vi "PathPlanner_Cmd_FollowRamsetePathExecute.vi"(5 "PathPlanner_Cmd_FollowRamConfig":T16={"ControlPastEnd_Sec"=3.0, "ReplanningConfig"={"enableInitialReplanning"=TRUE, "enableDynamicReplanning"=FALSE, "dynamicReplanningTotalErrorThreshold"=1.0, "dynamicReplanningErrorSpikeThreshold"=0.25}, "Trigger Events"=TRUE, "RAMSETE_EXE_TUNING SI"={"B"=2.0, "Zeta"=0.7, "X Tolerance M"=2.0, "Y Tolerance M"=0.7, "Heading Tolerance RAD"=0.7, "Track Width M"=2.0, "Max Speed M/S"=2.0}} {"RAMSETE_EXE_TUNING SI"."Max Speed M/S" format="%13.4f"; "RAMSETE_EXE_TUNING SI"."Track Width M" format="%13.4f"; "RAMSETE_EXE_TUNING SI"."Heading Tolerance RAD" format="%13.4f"; "RAMSETE_EXE_TUNING SI"."Y Tolerance M" format="%13.4f"; "RAMSETE_EXE_TUNING SI"."X Tolerance M" format="%13.4f"; "RAMSETE_EXE_TUNING SI"."Zeta" format="%13.4f"; "RAMSETE_EXE_TUNING SI"."B" format="%13.4f"}, 6 "PassthroughTime_SEC":dbl=-1.0, 7 "PathPlannerPath":T7={"BezierPoints"=[], "PreviewStartingRotation"={"VALUE"=0.0, "COS"=1.0, "SIN"=0.0}, "Reversed"=FALSE, "RotationTargets"=[], "ConstraintZones"=[], "EventMarkers"=[], "GlobalConstraints"={"MaxVelocityMps;"=0.0, "MaxAccelerationMpsSq;"=0.0, "MaxAngularVelRadPsEc;"=0.0, "MaxAngularAccRadPSecSq"=0.0, "Exists"=FALSE}, "GoalEndState"={"Velocity"=0.0, "Rotation"={"VALUE"=0.0, "COS"=1.0, "SIN"=0.0}}, "AllPoints"=[]} {"AllPoints"."HolonomicRotation"."SIN" format="%13.4f"; "AllPoints"."HolonomicRotation"."COS" format="%13.4f"; "AllPoints"."HolonomicRotation"."VALUE" format="%13.4f"; "AllPoints"."Position"."Y" format="%14.3f"; "AllPoints"."Position"."X" format="%14.3f"; "GoalEndState"."Rotation"."SIN" format="%13.4f"; "GoalEndState"."Rotation"."COS" format="%13.4f"; "GoalEndState"."Rotation"."VALUE" format="%13.4f"; "RotationTargets"."target"."SIN" format="%13.4f"; "RotationTargets"."target"."COS" format="%13.4f"; "RotationTargets"."target"."VALUE" format="%13.4f"; "PreviewStartingRotation"."SIN" format="%13.4f"; "PreviewStartingRotation"."COS" format="%13.4f"; "PreviewStartingRotation"."VALUE" format="%13.4f"; "BezierPoints"."Y" format="%14.3f"; "BezierPoints"."X" format="%14.3f"}, 8 "Enabled":bool=TRUE, 9 "Reset":bool, 10 "CurrentChassisSpeeds":T6 {"vOmega" format="%10.3f"; "vY" format="%10.3f"; "vX" format="%10.3f"}, 11 "Current Pose SI":T3={"TRANSLATION"={"X"=0.0, "Y"=0.0}, "ROTATION"={"VALUE"=0.0, "COS"=1.0, "SIN"=0.0}} {"ROTATION"."SIN" format="%13.4f"; "ROTATION"."COS" format="%13.4f"; "ROTATION"."VALUE" format="%13.4f"; "TRANSLATION"."Y" format="%14.3f"; "TRANSLATION"."X" format="%14.3f"}) -> (0 "Position Error M":dbl, 1 "Complete":bool, 2 "At Reference":bool, 3 "Left Right Speed Dmds":T1, 4 "outRAMSETE":T2={"B"=2.0, "Zeta"=0.7, "poseTolerance"={"TRANSLATION"={"X"=0.0, "Y"=0.0}, "ROTATION"={"VALUE"=0.0, "COS"=1.0, "SIN"=0.0}}, "poseError"={"TRANSLATION"={"X"=0.0, "Y"=0.0}, "ROTATION"={"VALUE"=0.0, "COS"=1.0, "SIN"=0.0}}, "Enabled"=TRUE} {"poseError"."ROTATION"."SIN" format="%13.4f"; "poseError"."ROTATION"."COS" format="%13.4f"; "poseError"."ROTATION"."VALUE" format="%13.4f"; "poseError"."TRANSLATION"."Y" format="%14.3f"; "poseError"."TRANSLATION"."X" format="%14.3f"; "poseTolerance"."ROTATION"."SIN" format="%13.4f"; "poseTolerance"."ROTATION"."COS" format="%13.4f"; "poseTolerance"."ROTATION"."VALUE" format="%13.4f"; "poseTolerance"."TRANSLATION"."Y" format="%14.3f"; "poseTolerance"."TRANSLATION"."X" format="%14.3f"; "Zeta" format="%12.3f"; "B" format="%12.3f"})   [LabVIEW 2019, in "PathPlanner24.lvlib"]
doc: "DOCUMENTATION IS NOT COMPLETE.\n \nCalculates the next output of the path following controller for holonomic drive robots. This wraps a Holonomic Drive Control function with the particulars needed to follow a PathPlanner trajectory.\n\nInputs:\n - PathPlanner_Holonomic_Ctrl_Pack_Tuning - cluster - The tuning paraameters for the holonomic drive controller. These are static. They should not be changed after the first call to this function.\n - CurrentPoseSi - pose2d - The current pose calculated by odometry or pose estimation. The pose can be absolute or relative depending on what type of trajectory is being followed.\n - PathPlannerState - cluster - The path palnner trajectory state containing the desired position and velocities of the robot.\n - Reset - boolean - When TRUE the holonomic drive controller is reset. This should be set to TRUE for the first execution of a trajectory.\n - Enabled - boolean - When TRUE, closed loop control is enabled. (Optional. Default: TRUE)\n - Period - double - The loop period in seconds for this controller. (Optional. Default: 0.020)\n\nOutputs:\n - CalcChassisSpeed - cluster - The desired chassis speed in SI units.\n - AtReference - boolean - TRUE if the robots position is within the defined tolerance.\n - PositionError - pose2d - Position error in SI units. How far the robot is away from the desired trajectory position.\n - out_Holonomic_Drive_Ctrl - THe current holonomic drive controller data cluster. This is mainly for diagnostic purposes."
uses:
  PathPlanner24.lvlib
  <vilib>/Rock Robotics/WPI/ThirdParty/JAS_Junk/TrajLib/TypeDef/POSE2D.ctl
  <vilib>/Rock Robotics/WPI/ThirdParty/JAS_Junk/TrajLib/TypeDef/TRANSLATION2D.ctl
  <vilib>/Rock Robotics/WPI/ThirdParty/JAS_Junk/TrajLib/TypeDef/ROTATION2D.ctl
  TypeDef/PathPlannerCmdFollowRamConfig.ctl
  TypeDef/PathPlannerReplanningConfig.ctl
  <vilib>/Rock Robotics/WPI/ThirdParty/JAS_Junk/TrajLib/TypeDef/RAMSETE_EXE_TUNING.ctl
  TypeDef/PathPlannerPath.ctl
  TypeDef/PathPlannerRotationTarget.ctl
  TypeDef/PathPlannerConstraintsZone.ctl
  TypeDef/PathPlannerPathConstraints.ctl
  TypeDef/PathPlannerEventMarker.ctl
  TypeDef/PathPlannerCommandUtil.ctl
  ENum/PathPlanner_CommandUtilType_ENUM.ctl
  TypeDef/PathPlannerGoalEndState.ctl
  TypeDef/PathPlannerPathPoint.ctl
  <vilib>/Rock Robotics/WPI/ThirdParty/JAS_Junk/TrajLib/TypeDef/CHASSIS_SPEEDS.ctl
  <vilib>/Rock Robotics/WPI/ThirdParty/JAS_Junk/TrajLib/TypeDef/RAMSETE.ctl
  PathPlanner_Cmd_Follow_Internal_InitEvents.vi
  PathPlanner_CommandUtil_Execute.vi
  <vilib>/Utility/error.llb/Clear Errors.vi
  <vilib>/Rock Robotics/WPI/ThirdParty/JAS_Junk/TrajLib/Trajectory_Library.lvlib
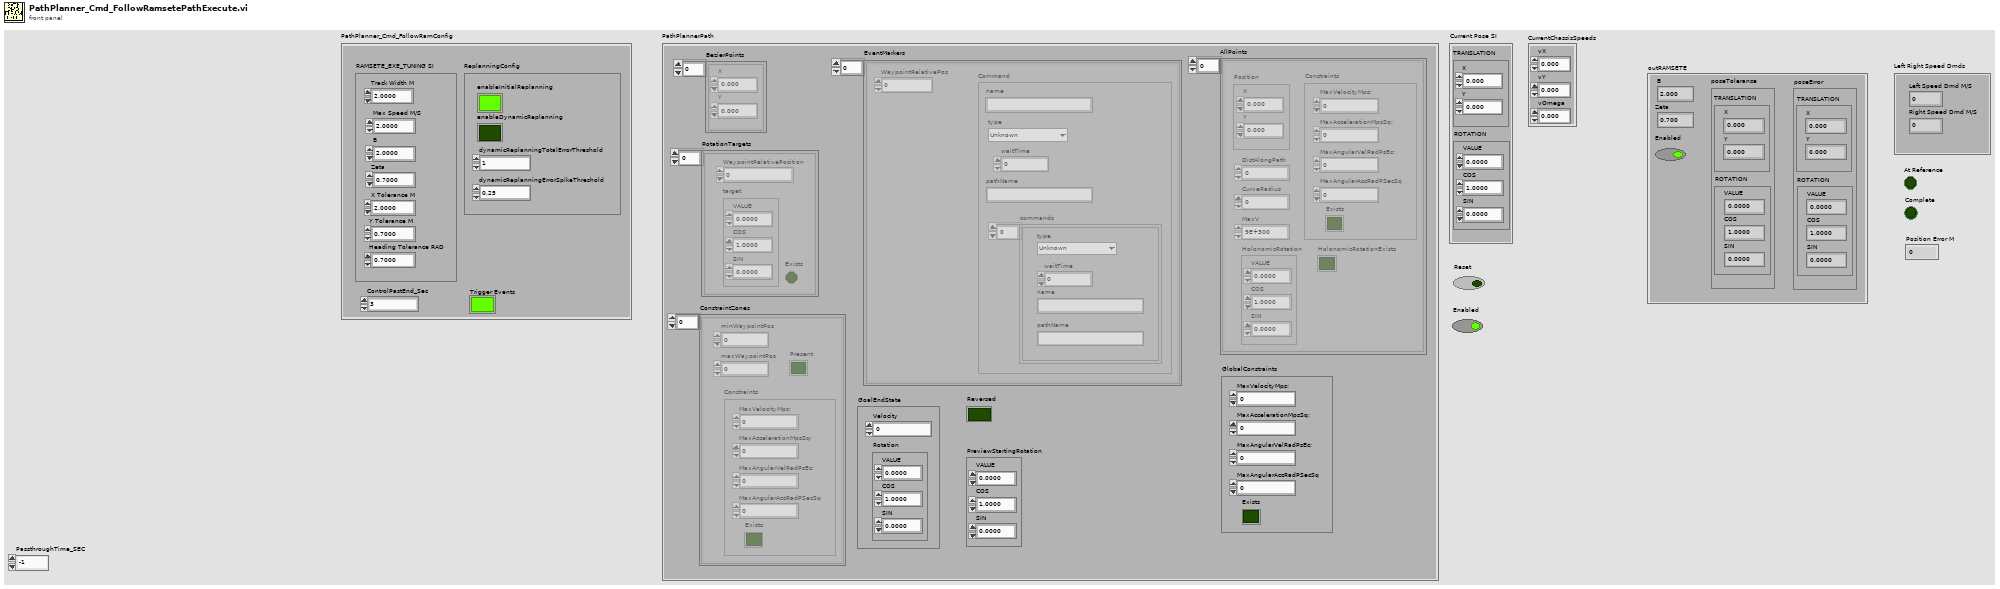
[diagram p1: front panel]
types:
  T1 = cluster{"Left Speed Dmd M/S":dbl, "Right Speed Dmd M/S":dbl}
  T2 = typedef "Trajectory_Library.lvlib/RAMSETE.ctl" = cluster{"B":dbl, "Zeta":dbl, "poseTolerance":T3, "poseError":T3, "Enabled":bool}
  T3 = typedef "Trajectory_Library.lvlib/POSE2D.ctl" = cluster{"TRANSLATION":T4, "ROTATION":T5}
  T4 = typedef "Trajectory_Library.lvlib/TRANSLATION2D.ctl" = cluster{"X":dbl, "Y":dbl}
  T5 = typedef "Trajectory_Library.lvlib/ROTATION2D.ctl" = cluster{"VALUE":dbl, "COS":dbl, "SIN":dbl}
  T6 = typedef "Trajectory_Library.lvlib/CHASSIS_SPEEDS.ctl" = cluster{"vX":dbl, "vY":dbl, "vOmega":dbl}
  T7 = typedef "PathPlanner24.lvlib/PathPlannerPath.ctl" = cluster{"BezierPoints":T4[], "PreviewStartingRotation":T5, "Reversed":bool, "RotationTargets":T8[], "ConstraintZones":T9[], "EventMarkers":T11[], "GlobalConstraints":T10, "GoalEndState":T14, "AllPoints":T15[]}
  T8 = typedef "PathPlanner24.lvlib/PathPlannerRotationTarget.ctl" = cluster{"target":T5, "WaypointRelativePosition":dbl, "Exists":bool}
  T9 = typedef "PathPlanner24.lvlib/PathPlannerConstraintsZone.ctl" = cluster{"minWaypointPos":dbl, "maxWaypointPos":dbl, "Constraints":T10, "Present":bool}
  T10 = typedef "PathPlanner24.lvlib/PathPlannerPathConstraints.ctl" = cluster{"MaxVelocityMps;":dbl, "MaxAccelerationMpsSq;":dbl, "MaxAngularVelRadPsEc;":dbl, "MaxAngularAccRadPSecSq":dbl, "Exists":bool}
  T11 = typedef "PathPlanner24.lvlib/PathPlannerEventMarker.ctl" = cluster{"WaypointRelativePos":dbl, "Command":T12}
  T12 = typedef "PathPlanner24.lvlib/PathPlannerCommandUtil.ctl" = cluster{"waitTime":dbl, "name":string, "pathName":string, "commands":cluster{"type":T13, "waitTime":dbl, "name":string, "pathName":string}[], "type":T13}
  T13 = typedef "PathPlanner24.lvlib/PathPlanner_CommandUtilType_ENUM.ctl" = enum16{"Unknown", "Wait", "Named", "Path", "Sequential", "Parallel", "Race", "Deadline"}
  T14 = typedef "PathPlanner24.lvlib/PathPlannerGoalEndState.ctl" = cluster{"Velocity":dbl, "Rotation":T5}
  T15 = typedef "PathPlanner24.lvlib/PathPlannerPathPoint.ctl" = cluster{"Position":T4, "HolonomicRotation":T5, "DistAlongPath":dbl, "CurveRadius":dbl, "MaxV":dbl, "Constraints":T10, "HolonomicRotationExists":bool}
  T16 = typedef "PathPlanner24.lvlib/PathPlannerCmdFollowRamConfig.ctl" = cluster{"ControlPastEnd_Sec":dbl, "ReplanningConfig":T17, "Trigger Events":bool, "RAMSETE_EXE_TUNING SI":T18}
  T17 = typedef "PathPlanner24.lvlib/PathPlannerReplanningConfig.ctl" = cluster{"enableInitialReplanning":bool, "enableDynamicReplanning":bool, "dynamicReplanningTotalErrorThreshold":dbl, "dynamicReplanningErrorSpikeThreshold":dbl}
  T18 = typedef "Trajectory_Library.lvlib/RAMSETE_EXE_TUNING.ctl" = cluster{"B":dbl, "Zeta":dbl, "X Tolerance M":dbl, "Y Tolerance M":dbl, "Heading Tolerance RAD":dbl, "Track Width M":dbl, "Max Speed M/S":dbl}
  T19 = cluster{"Traj Time Plus Extra\nElapsed":bool, "Traj Time Elapsed":bool}
  T20 = typedef "PathPlanner24.lvlib/PathPlannerTrajectoryState.ctl" = cluster{"TimeSeconds":dbl, "VelocityMPS":dbl, "AccerationMpsSq":dbl, "HeadingAngularVelRadPerSec":dbl, "PositionMeters":T4, "Heading":T5, "TargetHolonomicRotation":T5, "CurvatureRadPerMeter":dbl, "PathPlannerConstraints":T10, "DeltaPos":dbl}
  T21 = typedef "PathPlanner24.lvlib/PathPlannerTrajectoryEvents.ctl" = cluster{"EventCommands":T22[]}
  T22 = typedef "PathPlanner24.lvlib/PathPlannerTrajectoryEvent.ctl" = cluster{"TimeStampSec":dbl, "CommandUtil":T12}
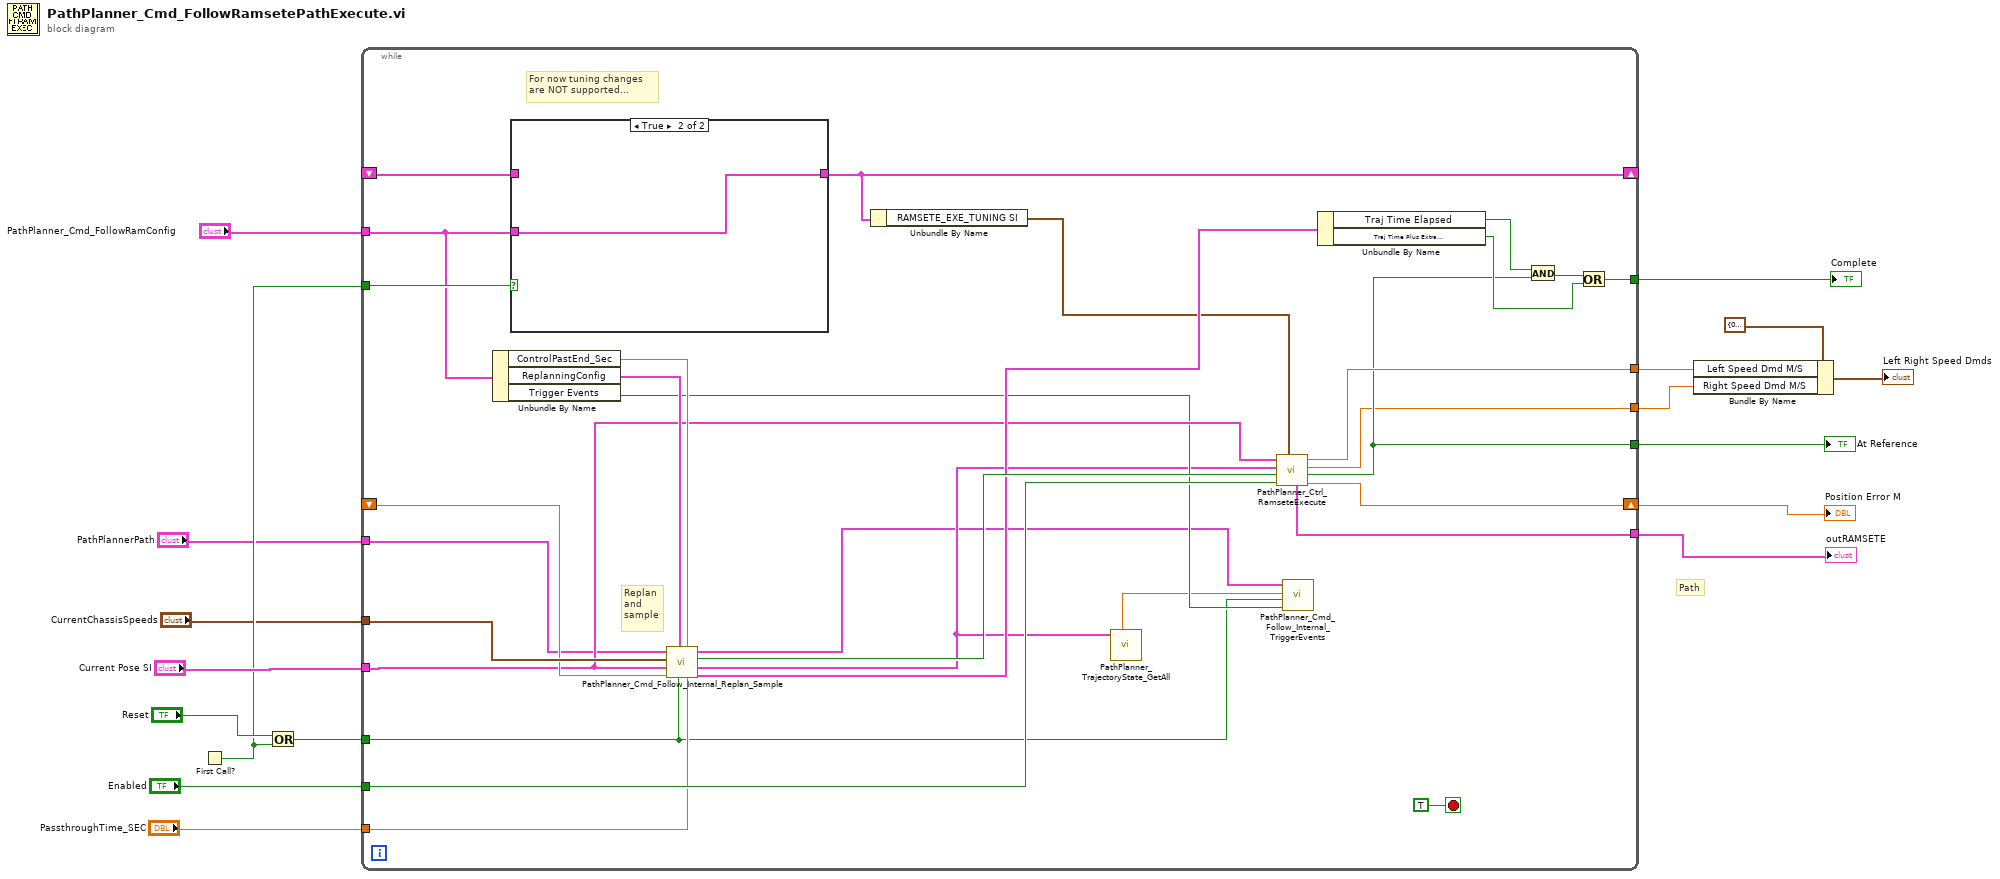
[diagram p0: block diagram]
diagram:
  # "Path"
  n1 = First Call?() -> (First Call?: T/F=w11:bool)
  n2 = Or(x="Reset", y=w11) -> (x .or. y?=w13:bool)
  n3 = while {
    tunnel: "PathPlanner_Cmd_FollowRamConfig" -> [w37]
    tunnel: "Current Pose SI" -> [w24]
    tunnel: w11 -> [w47]
    shift-right: [w26] -> _
    shift-left: _ -> [w45]
    tunnel: "Enabled" -> [w44]
    tunnel: [w29] -> w12
    tunnel: "CurrentChassisSpeeds" -> [w40]
    tunnel: "PassthroughTime_SEC" -> [w39]
    tunnel: [w42] -> w5
    shift-right: [w43] -> w9
    shift-left: _ -> [w38]
    tunnel: w13 -> [w19]
    tunnel: "PathPlannerPath" -> [w20]
    tunnel: [w34] -> w6
    tunnel: [w30] -> w2
    tunnel: [w28] -> w1
    stop <- TRUE stop-if-true
    # "Replan\nand \nsample"
    # "For now tuning changes\nare NOT supported..."
    n4 = Unbundle By Name(w37) -> ("ControlPastEnd_Sec"=w27:dbl, "ReplanningConfig"=w36:T17, "Trigger Events"=w23:bool)
    n5 = case shown="True" w47 {
      tunnel: [w48 w49] -> w26
      tunnel: w37 -> [_ w49]
      tunnel: w45 -> [w48 _]
      frame False {
      }
      frame True {
      }
    }
    n6 = call "PathPlanner_Cmd_Follow_Internal_Replan_Sample.vi"("PassthroughTime_SEC"=w39, "Extra Time Sec"=w27, "Reset In"=w19, "ReplanningConfig"=w36, "Position Error M"=w38, "Current Pose SI"=w24, "CurrentChassisSpeeds"=w40, "RePlannedPath in"=w20) -> ("Traj End Status"=w33:T19, "Trajectory State"=w22:T20, "Reset Controller"=w41:bool, "PathPlannerTrajectoryEvents"=w18:T21)
    n7 = Unbundle By Name(w26) -> ("RAMSETE_EXE_TUNING SI"=w25:T18)
    n8 = call "PathPlanner_TrajectoryState_GetAll.vi"("PathPlannerState"=w22) -> ("TimeSeconds"=w21:dbl)  [unwired: 1 in, 9 out]
    n9 = call "PathPlanner_Ctrl_RamseteExecute.vi"("RAMSETE_EXE_TUNING SI"=w25, "Enabled"=w44, "Reset"=w41, "PathPlannerState"=w22, "Current Pose SI"=w24) -> ("Position Error M"=w43:dbl, "At Reference"=w29:bool, "Right Speed Dmd M/S"=w28:dbl, "Left Speed Dmd M/S"=w30:dbl, "outRAMSETE"=w42:T2)  [unwired: 2 in]
    n10 = call "PathPlanner_Cmd_Follow_Internal_TriggerEvents.vi"("TrigerEvents"=w23, "Reset"=w19, "TrajectoryTimeStampSecs"=w21, "PathPlannerTrajectoryEvents"=w18) -> ()  [unwired: 8 in]
    n11 = Unbundle By Name(w33) -> ("Traj Time Elapsed"=w32:bool, "Traj Time Plus Extra\nElapsed"=w31:bool)
    n12 = And(x=w32, y=w29) -> (x .and. y?=w35:bool)
    n13 = Or(x=w35, y=w31) -> (x .or. y?=w34:bool)
  }
  "At Reference" <- w12
  "Position Error M" <- w9
  "Complete" <- w6
  "outRAMSETE" <- w5
  n14 = Bundle By Name(cluster=T1 {"Left Speed Dmd M/S"=0.0, "Right Speed Dmd M/S"=0.0} ("Left Right Speed Dmds"), "Left Speed Dmd M/S"=w2, "Right Speed Dmd M/S"=w1) -> (→"Left Right Speed Dmds":T1)
